vi "Forward Substatus to Parent.vi"(8 "error in (no error)":errorcluster, 10 "Module Substatus":T1, 11 "Module in":refnum<class "Module.lvclass">) -> (0 "error out":errorcluster, 3 "Module out":refnum<class "Module.lvclass">)   [LabVIEW 2020, in "Volatus.lvlib" / "Module.lvclass"]
uses:
  Module.lvclass
  Module.lvclass/Module.ctl
  MessageQ/MessageQ.lvclass
  Module Substatus.ctl
  Volatus.lvlib
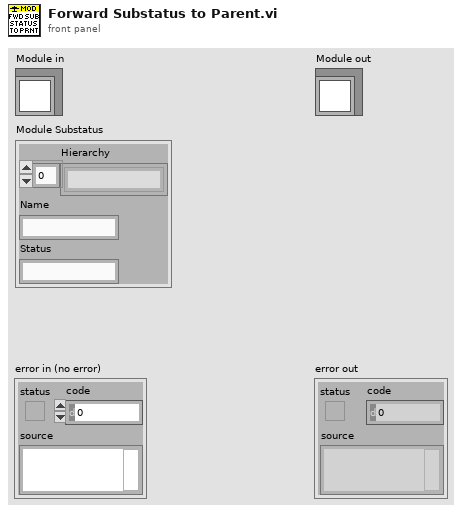
[diagram p1: front panel]
types:
  T1 = typedef "Volatus.lvlib/Module Substatus.ctl" = cluster{"Hierarchy":string[], "Name":string, "Status":string}
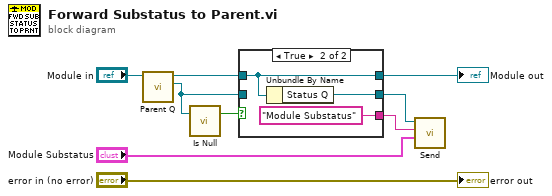
[diagram p0: block diagram]
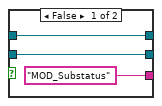
[diagram p2: hidden frame]
diagram:
  n1 = call "Parent Q.vi"("Module in"="Module in") -> ("Parent Q"=w6:refnum<class "MessageQ.lvclass">, "Module out"=w2:refnum<class "Module.lvclass">)  [unwired: 9 in]
  n2 = call "Is Null.vi"("MessageQ in"=w6) -> ("Null"=w7:bool)  [unwired: 2 in]
  n3 = case shown="True" w7 {
    tunnel: w6 -> [w11 _]
    tunnel: ["MOD_Substatus" ("ID") "Module Substatus" ("ID")] -> w4
    tunnel: [w11 w13] -> w3
    tunnel: w2 -> [w10 w14]
    tunnel: [w10 w14] -> w1
    frame False {
    }
    frame True {
      n4 = Unbundle By Name(w14) -> ("Status Q"=w13:refnum<class "MessageQ.lvclass">)
    }
  }
  "Module out" <- w1
  n5 = call "Send.vi"("Data"="Module Substatus", "ID"=w4, "MessageQ in"=w3) -> ()  [unwired: 7 in, 2 out]
  "error out" <- "error in (no error)"
